vi "read_data_feed_single_use(SubVI).vi"(8 "error in (no error)":errorcluster) -> (0 "error out":errorcluster, 3 "appended array":dbl[](array[numeric]))   [LabVIEW 2014]
uses:
  <vilib>/xml/Load XML String.vi
  <vilib>/xml/Close Reference(Node).vi
  Program Files (x86)/National Instruments/LabVIEW 2014/vi.lib/addons/internet/NI_InternetTK_Core_VIs.lvlib
  <vilib>/xml/NI_XML.lvlib
  <resource>/objmgr/DOMUserDefRef.rc
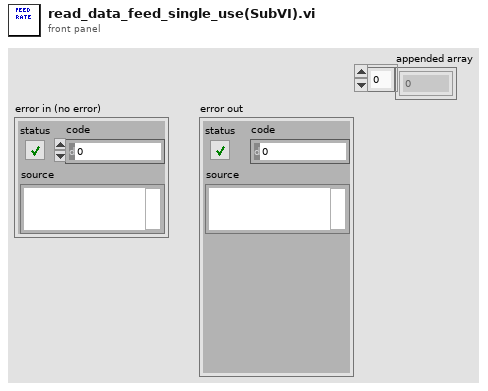
[diagram p1: front panel]
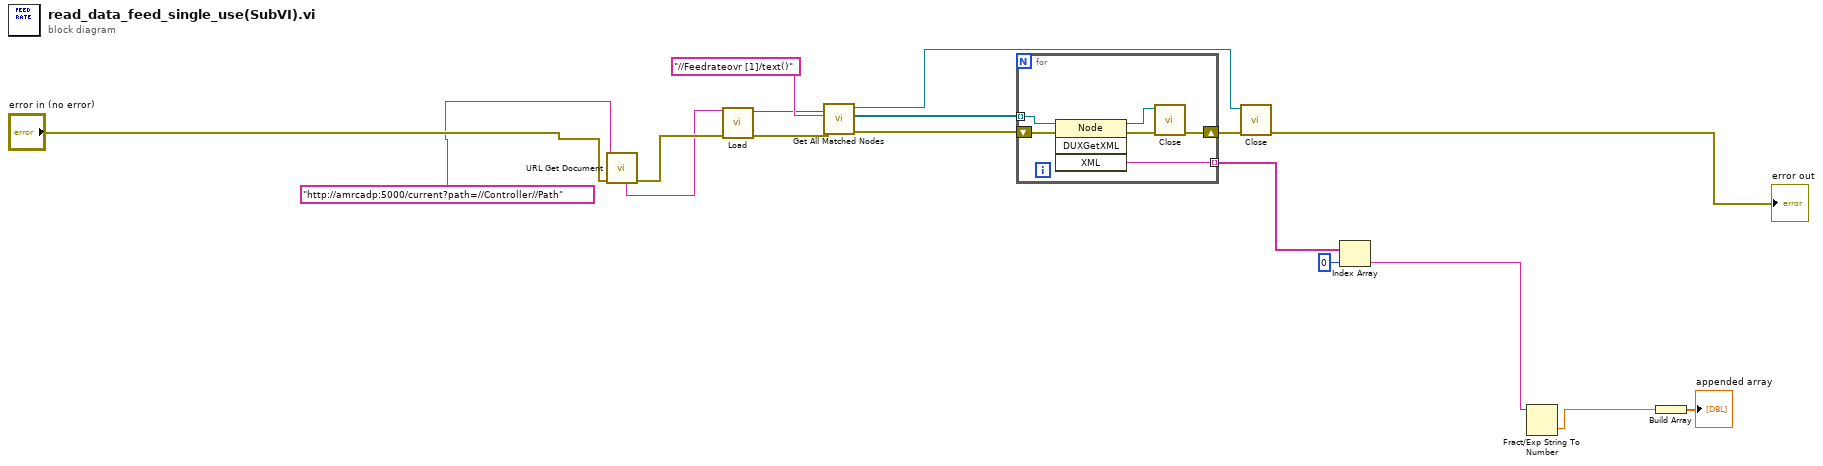
[diagram p0: block diagram]
diagram:
  n1 = call "URL Get Document.vi"("error in (no error)"="error in (no error)", "URL"="http://amrcadp:5000/current?path=//Controller//Path") -> ("error out"=w15:errorcluster, "content"=w12:string)  [unwired: 5 in, 3 out]
  n2 = call-poly <vilib>:"Load.vi"("XML string"=w12, "error in (no error)"=w15) -> ("DOM document out"=w9:refnum<k20>, "error out"=w10:errorcluster)  [unwired: 11 in, 1 out]
  n3 = call <vilib>:"Get All Matched Nodes.vi"("error in (no error)"=w10, "XPath expression"="//Feedrateovr [1]/text()", "node in"=w9) -> ("error out"=w7:errorcluster, "node result array"=w6:refnum<k20>[], "node out"=w11:refnum<k20>)  [unwired: 6 out]
  n4 = for {
    tunnel: w6 -> [w19] mode=indexing
    shift-right: [w21] -> w8
    shift-left: w7 -> [w20]
    tunnel: [w18] -> w5 mode=indexing
    n5 = invoke on="Invoke Node" class="Node" method="DUXGetXML"(reference=w19, error in=w20) -> (reference out=w22:refnum<k20>, error out=w23:errorcluster, "XML"=w18:string)  [unwired: 2 in, 1 out]
    n6 = call-poly <vilib>:"Close.vi"("error in (no error)"=w23, "node"=w22) -> ("error out"=w21:errorcluster)  [unwired: 7 out]
  }
  n7 = call-poly <vilib>:"Close.vi"("error in (no error)"=w8, "node"=w11) -> ("error out"=→"error out":errorcluster)  [unwired: 7 out]
  n8 = Index Array(array=w5, index=0) -> (element=w3:string)
  n9 = Fract/Exp String To Number(string=w3) -> (number=w2:dbl)  [unwired: 3 in, 1 out]
  n10 = Build Array(w2) -> (→"appended array":dbl[])
